vi "niFpgaScaledWinOutsideSCTLIndex.vi"(0 "real data in":fxp<+/-,24,1>, 5 "imaginary data in":fxp<+/-,24,1>, 7 "coefficient index":u16) -> (3 "data index":u16, 4 "real data out":fxp<+/-,24,-1>, 6 "imaginary data out":fxp<+/-,24,-1>)   [LabVIEW 2017]
uses:
  <vilib>/Platform/TimedLoop/XDataNode/timing_clust.ctl
  <vilib>/Platform/TimedLoop/XDataNode/nitl_modes.ctl
  <vilib>/Platform/TimedLoop/XDataNode/wakeup.ctl
  <vilib>/Platform/TimedLoop/XDataNode/XDataNode.xnode
  <vilib>/rvi/FXPMathLib/FxpMul/XNode/nifxpmath_Multiplier.xnode
  <vilib>/Platform/TimedLoop/XDataNode/XDNodeRunTimeDep.lvlib
  <vilib>/rvi/FXPMathLib/sim/FxpSim.dll
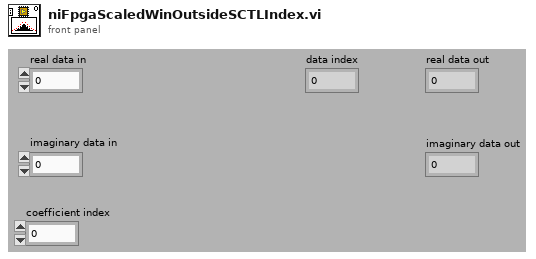
[diagram p1: front panel]
types:
  T1 = typedef "XDNodeRunTimeDep.lvlib/timing_clust.ctl" = cluster{"Expected End [f-1]":u64, "Actual End [f-1]":u64, "Finished Late? [f-1]":bool, "Expected End [i-1]":u64, "Actual End [i-1]":u64, "Finished Late? [i-1]":bool, "Expected Start [i]":u64, "Actual Start [i]":u64, "Expected Start [f]":u64, "Actual Start [f]":u64, "Source Name":string, "Structure Name":string, "Period":i64, "Deadline":i64, "Offset":i64, "Start":i64, "Priority":i32, "Timeout":i32, "Mode":T2, "Wakeup Reason":T3, "Error":errorcluster, "Source Type":string, "Secondary Source Type":string, "Global End Time":u64, "Global Start Time":u64, "Frame Duration":u64, "Iteration Duration":u64, "Assigned CPU":i32, "I/O Scan Engine Mode":u32}
  T2 = typedef "XDNodeRunTimeDep.lvlib/nitl_modes.ctl" = enum32{"No Change", "Process missed periods, maintain original phase", "Discard missed periods, maintain original phase", "Process missed periods, ignore original phase", "Discard missed periods, ignore original phase"}
  T3 = typedef "XDNodeRunTimeDep.lvlib/wakeup.ctl" = enum32{"Normal", "Aborted", "Asynchronous wakeup", "Timing source error", "Timed loop error", "Timeout"}
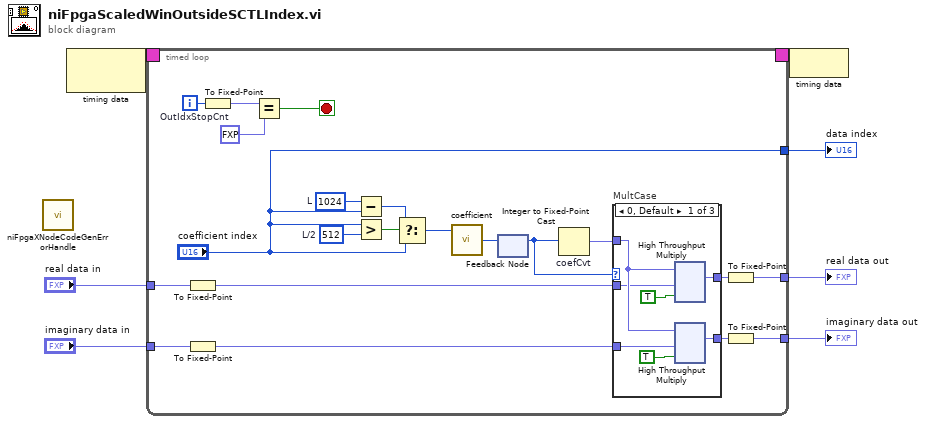
[diagram p0: block diagram]
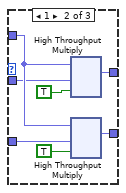
[diagram p2: hidden frame]
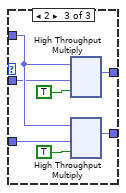
[diagram p3: hidden frame]
diagram:
  n1 = call <vilib>:"niFpgaXNodeCodeGenErrorHandle.vi"() -> ()  [unwired: 1 in]
  n2 = node-c288() -> (w2:T1)  [unwired: 1 out]
  n3 = timed-loop "MainLoop" {
    tunnel: "real data in" -> [w14]
    tunnel: "imaginary data in" -> [w13]
    tunnel: ["coefficient index"] -> w4
    timing: w2 -> [_]
    timing-out: [_] -> w1
    tunnel: [w16] -> w6
    tunnel: [w15] -> w3
    i -> [w27]
    stop <- w19 stop-if-true
    w12 = fxp<+,3,3> 2.0  # OutIdxStopCnt
    w24 = u16 1024  # L
    w26 = u16 512  # L/2
    n4 = To Fixed-Point(number=w14) -> (fixed-point=w11:fxp<+/-,24,1>)  [unwired: 1 in]
    n5 = To Fixed-Point(number=w13) -> (fixed-point=w10:fxp<+/-,24,1>)  [unwired: 1 in]
    n6 = To Fixed-Point(number=w27) -> (fixed-point=w20:fxp<+,3,3>)  [unwired: 1 out]
    n7 = Equal?(x=w20, y=w12) -> (x = y?=w19:bool)
    n8 = Subtract(x=w24, y="coefficient index") -> (x-y=w25:u16)
    n9 = Greater?(x="coefficient index", y=w26) -> (0:w28:bool)
    n10 = Select(t=w25, s=w28, f="coefficient index") -> (s? t:f=w22:u16)
    n11 = call "coefficient"("address"=w22) -> ("data out"=w23:i32)  [unwired: 8 in]
    n12 = feedback-in #1(w23) -> ()
    n13 = feedback #1() -> (w9:i32)  [unwired: 1 out]
    n14 = Integer to Fixed-Point Cast "coefCvt"(integer=w9) -> (fixed-point=w8:fxp<+/-,32,32>)  [unwired: 1 in]
    n15 = case "MultCase" shown="0, Default" w9 {
      tunnel: [w35 w42 w49] -> w18
      tunnel: [w34 w41 w48] -> w17
      tunnel: w8 -> [w33 w40 w47]
      tunnel: w11 -> [w30 w37 w44]
      tunnel: w10 -> [w29 w36 w43]
      frame 0, Default {
        n16 = xnode "High Throughput Multiply"("x"=w33, "y"=w30, "input valid"=TRUE) -> ("x*y"=w35:fxp<+/-,56,33>)  [unwired: 1 in, 2 out]
        n17 = xnode "High Throughput Multiply"("x"=w33, "y"=w29, "input valid"=TRUE) -> ("x*y"=w34:fxp<+/-,56,33>)  [unwired: 1 in, 2 out]
      }
      frame 1 {
        n18 = xnode "High Throughput Multiply"("x"=w40, "y"=w37, "input valid"=TRUE) -> ("x*y"=w42:fxp<+/-,56,33>)  [unwired: 1 in, 2 out]
        n19 = xnode "High Throughput Multiply"("x"=w40, "y"=w36, "input valid"=TRUE) -> ("x*y"=w41:fxp<+/-,56,33>)  [unwired: 1 in, 2 out]
      }
      frame 2 {
        n20 = xnode "High Throughput Multiply"("x"=w47, "y"=w44, "input valid"=TRUE) -> ("x*y"=w49:fxp<+/-,56,33>)  [unwired: 1 in, 2 out]
        n21 = xnode "High Throughput Multiply"("x"=w47, "y"=w43, "input valid"=TRUE) -> ("x*y"=w48:fxp<+/-,56,33>)  [unwired: 1 in, 2 out]
      }
    }
    n22 = To Fixed-Point ("MultCast")(number=w18) -> (fixed-point=w16:fxp<+/-,24,-1>)  [unwired: 1 out]
    n23 = To Fixed-Point ("MultCast")(number=w17) -> (fixed-point=w15:fxp<+/-,24,-1>)  [unwired: 1 out]
  }
  "data index" <- w4
  "real data out" <- w6
  "imaginary data out" <- w3
  n24 = node-c288(w1) -> ()
